vi "CameraSetTimeout.vi"(8 "error in (no error)":errorcluster, 10 "Timeout":u32, 11 "CameraBase in":refnum<class "CameraBase.lvclass">) -> (0 "error out":errorcluster, 2 "Timeout set":u32, 3 "CameraBase out":refnum<class "CameraBase.lvclass">)   [LabVIEW 2010, in "CameraBase.lvclass"]
uses:
  CameraBase.lvclass
panel:
  # "Camera Configuration"
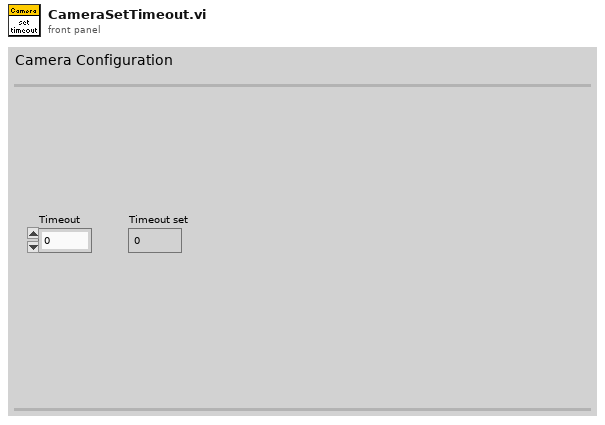
[diagram p1: front panel]
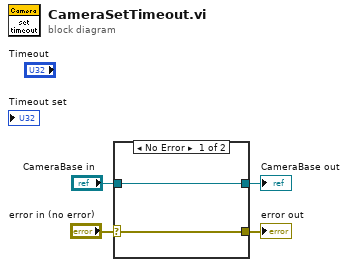
[diagram p0: block diagram]
diagram:
  n1 = case shown="No Error" "error in (no error)" {
    selector: "error in (no error)" -> [w6 w8]
    tunnel: [w6 w8] -> w4
    tunnel: [w5 w7] -> w3
    tunnel: "CameraBase in" -> [w5 w7]
    frame No Error {
    }
    frame Error {
    }
  }
  "error out" <- w4
  "CameraBase out" <- w3
